vi "Feeder Position.vi"(2 "setpoint":dbl format="%.2f", 3 "Z Axis":dbl) -> (0 "Rate":dbl, 1 "Finished":bool)   [LabVIEW 2012]
uses:
  <vilib>/addons/control/pid/pid.llb/PID (DBL).vi
  <vilib>/addons/control/pid/NI_PID_pid.lvlib
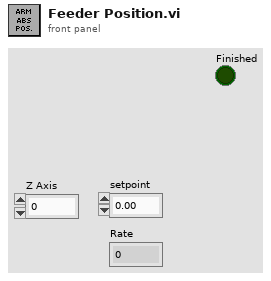
[diagram p1: front panel]
types:
  T1 = cluster{"proportional gain (Kc)":dbl, "integral time (Ti, min)":dbl, "derivative time (Td, min)":dbl}
  T2 = typedef "WPI_EncoderDevRef.ctl" = cluster{"DevStatus":errorcluster, "EncoderIndex":T3, "CounterIndex":T4, "DistancePerCount":dbl, "Decoding Type":T5}
  T3 = typedef "FPGA_EncoderIdx.ctl" = enum8{"Enc 0", "Enc 1", "Enc 2", "Enc 3", "Invalid"}
  T4 = typedef "FPGA_CounterCtrSystemIndex.ctl" = enum8{"Ctr 0", "Ctr 1", "Ctr 2", "Ctr 3", "Ctr 4", "Ctr 5", "Ctr 6", "Ctr 7", "Invalid"}
  T5 = typedef "WPI_EncoderType.ctl" = enum16{"1x", "2x", "4x"}
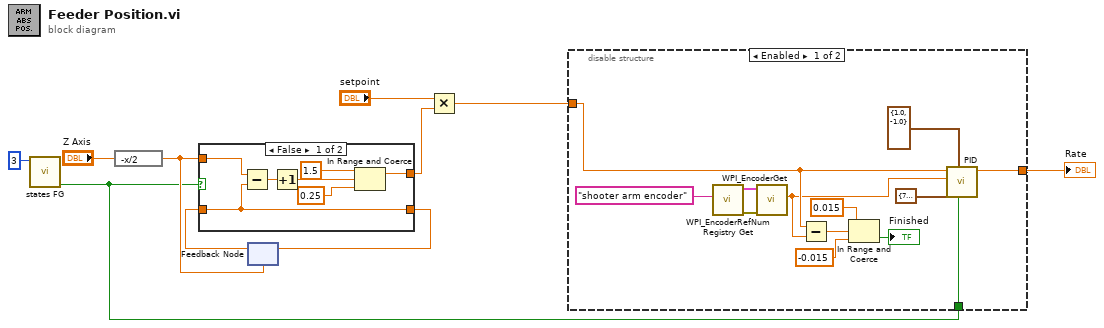
[diagram p0: block diagram]
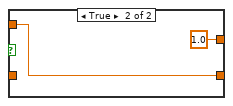
[diagram p2: hidden frame]
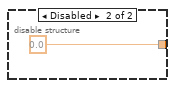
[diagram p3: hidden frame]
diagram:
  n1 = call "states FG.vi"("Loop ID"=3) -> ("first call?"=w1:bool)  [unwired: 7 in, 3 out]
  n2 = expression code="-x/2"("Z Axis") -> (w2:dbl)
  n3 = feedback #1(w2) -> (w6:dbl)
  n4 = case shown="False" w1 {
    tunnel: w2 -> [w17 w19]
    tunnel: [w16 w19] -> w7
    tunnel: w6 -> [w16 _]
    tunnel: [w13 1.0 ("upper limit")] -> w5
    frame False {
      n5 = Subtract(x=w17, y=w16) -> (x-y=w12:dbl)
      n6 = Increment(x=w12) -> (x+1=w11:dbl)
      n7 = In Range and Coerce(upper limit=1.5, x=w11, lower limit=0.25) -> (coerced(x)=w13:dbl)  [unwired: 1 out]
    }
    frame True {
    }
  }
  n8 = feedback-in #1(w7) -> ()
  n9 = Multiply(x="setpoint", y=w5) -> (x*y=w8:dbl)
  n10 = disable-structure shown="Enabled" {
    disable-tunnel: [w28 0.0 ("Rate")] -> w10
    disable-tunnel: w8 -> [w25 _]
    disable-tunnel: w1 -> [w26 _]
    frame Enabled {
      n11 = call <vilib>:"WPI_EncoderRefNum Registry Get.vi"("refnum name"="shooter arm encoder") -> ("error out"=w32:errorcluster, "EncoderDevRef"=w31:T2)  [unwired: 9 in]
      n12 = call <vilib>:"WPI_EncoderGet.vi"("error in (no error)"=w32, "EncoderDevRef"=w31) -> ("Distance"=w24:dbl)  [unwired: 4 in, 5 out]
      n13 = Subtract(x=w25, y=w24) -> (x-y=w23:dbl)
      n14 = In Range and Coerce(upper limit=0.015, x=w23, lower limit=-0.015) -> (In Range?=→"Finished":bool)  [unwired: 1 out]
      n15 = call-poly <vilib>:"PID.vi"("reinitialize? (F)"=w26, "output range"=cluster{"output high":dbl, "output low":dbl} {"output high"=1.0, "output low"=-1.0}, "PID gains"=T1 {"proportional gain (Kc)"=7.0, "integral time (Ti, min)"=0.01, "derivative time (Td, min)"=0.0}, "process variable"=w24, "setpoint"=w25) -> ("output"=w28:dbl)  [unwired: 5 in, 1 out]
    }
    frame Disabled {
    }
  }
  "Rate" <- w10
